vi "Send Command.vi"(8 "error out (no error)":errorcluster, 10 "Command":string, 11 "VISA resource name in":refnum<visa-resource-name>) -> (0 "error out":errorcluster, 3 "VISA resource name out":refnum<visa-resource-name>)   [LabVIEW 2015]
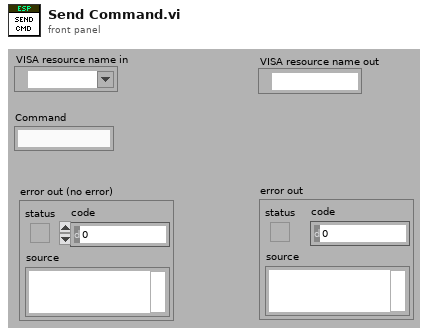
[diagram p1: front panel]
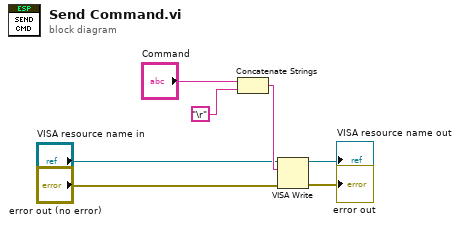
[diagram p0: block diagram]
diagram:
  n1 = Concatenate Strings("Command", "\r") -> (w7:string)
  n2 = VISA Write(VISA resource name="VISA resource name in", write buffer=w7, error in (no error)="error out (no error)") -> (VISA resource name out=→"VISA resource name out":refnum<visa-resource-name>, error out=→"error out":errorcluster)  [unwired: 1 out]
